vi "Pipe Var Intf - Read Variable - Complex Double.vi"(8 "error in (no error)":errorcluster, 9 "max dims (0: scalar)":i32, 10 "variable name":string, 11 "GOLPI ref. in":T1={"pipe handle"={"lv_proc.dll file path"=path "", "process instance handle"=[], "debug mode"=FALSE, "debug data"=[]}, "fast read timeout [ms]"=500, "fast read settle time [ms]"=10, "fast read to multiple [ms]"=1, "max elements per input line"=100, "slow read timeout [ms]"=5000, "stdin double format specifier"="%_16e", "max elements per stdout output column"=100, "console mode bitstream"=FALSE, "bitstream first read timeout [ms]"=1000, "bitstream read timeout [ms]"=50, "struct transfer possible"=FALSE, "matlab mode"=FALSE, "var pipe write timeout [ms]"=5000, "variable pipe mode"=FALSE, "variable pipe buffer size [Bytes]"=10000000, "variable pipe block size [Bytes]"=1000000} {"variable pipe block size [Bytes]" format="%.0p"; "variable pipe buffer size [Bytes]" format="%.0p"}) -> (0 "error out":errorcluster, 2 "data out":cdb[][](array[numeric]), 3 "GOLPI ref. out":T1={"pipe handle"={"lv_proc.dll file path"=path "", "process instance handle"=[], "debug mode"=FALSE, "debug data"=[]}, "fast read timeout [ms]"=500, "fast read settle time [ms]"=10, "fast read to multiple [ms]"=1, "max elements per input line"=100, "slow read timeout [ms]"=5000, "stdin double format specifier"="", "max elements per stdout output column"=100, "console mode bitstream"=FALSE, "bitstream first read timeout [ms]"=1000, "bitstream read timeout [ms]"=50, "struct transfer possible"=FALSE, "matlab mode"=FALSE, "var pipe write timeout [ms]"=5000, "variable pipe mode"=FALSE, "variable pipe buffer size [Bytes]"=10000000, "variable pipe block size [Bytes]"=1000000} {"variable pipe block size [Bytes]" format="%.0p"; "variable pipe buffer size [Bytes]" format="%.0p"})   [LabVIEW 2020, in "GOLPI library.lvlib"]
doc: "Read matrix from Octave using pipe variable interface. In case of compatible non-doubles, casts to double. max dims defines maximum expected dimensions count."
uses:
  GOLPI library.lvlib
  Public/GOLPI reference Type Def.ctl
  LV Process source distribution/Pipe Handle.ctl
  <vilib>/Utility/error.llb/Error Cluster From Error Code.vi
  <vilib>/ErrorRing/Error Ring.xnode
  LV Process source distribution/LV Process library.lvlib
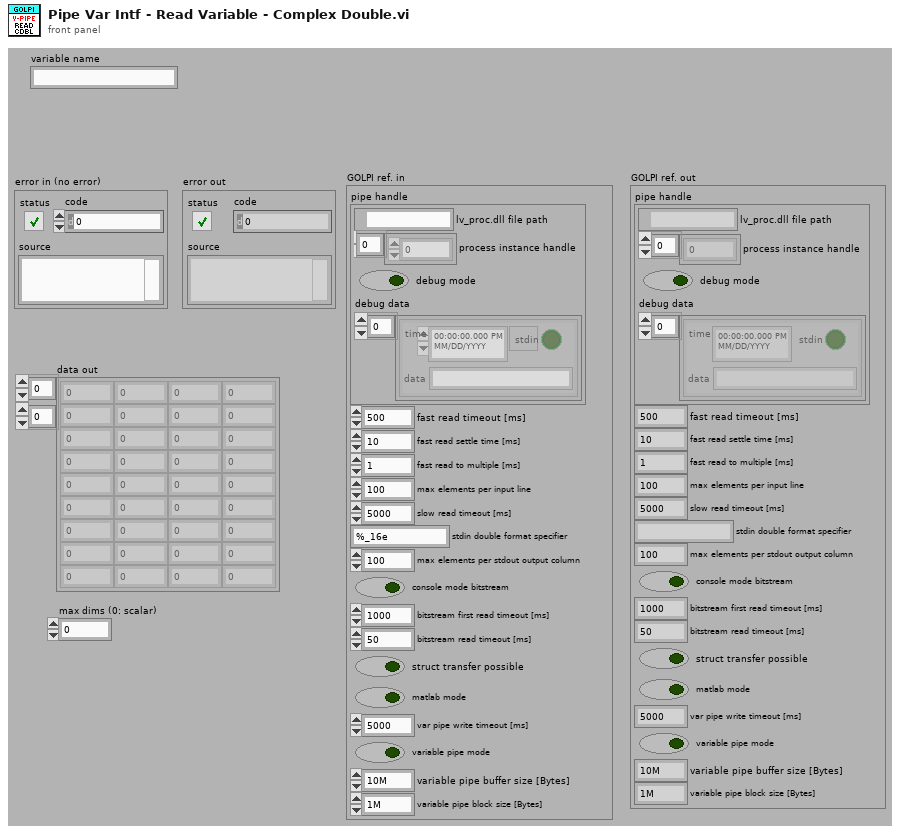
[diagram p1: front panel]
types:
  T1 = typedef "GOLPI library.lvlib/GOLPI reference Type Def.ctl" = cluster{"pipe handle":T2, "fast read timeout [ms]":u32, "fast read settle time [ms]":u32, "fast read to multiple [ms]":u32, "max elements per input line":u32, "slow read timeout [ms]":u32, "stdin double format specifier":string, "max elements per stdout output column":u32, "console mode bitstream":bool, "bitstream first read timeout [ms]":u32, "bitstream read timeout [ms]":u32, "struct transfer possible":bool, "matlab mode":bool, "var pipe write timeout [ms]":u32, "variable pipe mode":bool, "variable pipe buffer size [Bytes]":u32, "variable pipe block size [Bytes]":u32}
  T2 = typedef "LV Process library.lvlib/Pipe Handle.ctl" = cluster{"lv_proc.dll file path":path, "process instance handle":u32[], "debug mode":bool, "debug data":cluster{"time":timestamp, "stdin":bool, "data":string}[]}
  T3 = typedef "GOLPI library.lvlib/Pipe Var Intf - Data Type.ctl" = enum16{"error", "String", "int32", "uint32", "double", "cplx double", "single", "cplx single"}
  T4 = enum16{"big-endian, network order", "native, host order", "little-endian"}
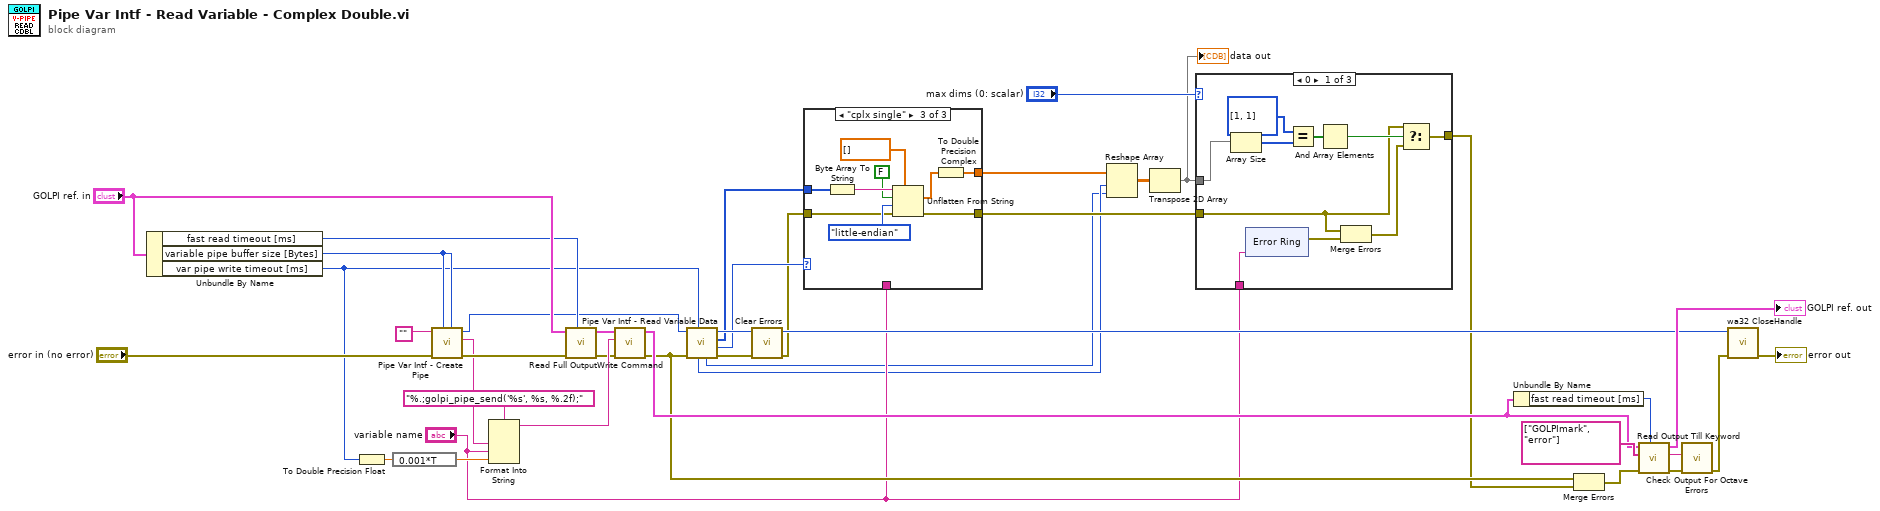
[diagram p0: block diagram]
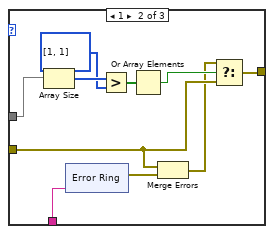
[diagram p2: hidden frame]
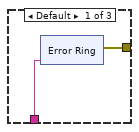
[diagram p4: hidden frame]
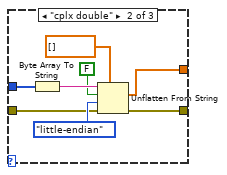
[diagram p5: hidden frame]
diagram:
  n1 = Unbundle By Name("GOLPI ref. in") -> ("fast read timeout [ms]"=w21:u32, "variable pipe buffer size [Bytes]"=w36:u32, "var pipe write timeout [ms]"=w16:u32)
  n2 = To Double Precision Float(number=w16) -> (double precision float=w34:dbl)
  n3 = expression code="0.001*T"(w34) -> (w35:dbl)
  n4 = call "Pipe Var Intf - Create Pipe.vi"("outBufferSize (256k)"=w36, "inBufferSize (256k)"=w36, "error in (no error)"="error in (no error)", "pipe name in (leave empty to generate random name)"="") -> ("error out"=w24:errorcluster, "pipe name out"=w18:string, "pipe handle out"=w17:i32)  [unwired: 5 in]
  n5 = Format Into String(format string="%.;golpi_pipe_send('%s', %s, %.2f);", w18, "variable name", w35) -> (resulting string=w38:string)  [unwired: 2 in, 1 out]
  n6 = call "Read Full Output.vi"("timeout [ms]"=w21, "error in"=w24, "GOLPI ref. in"="GOLPI ref. in") -> ("error out"=w25:errorcluster, "GOLPI ref. out"=w22:T1)  [unwired: 5 in, 2 out]
  n7 = call "Write Command.vi"("error in"=w25, "command"=w38, "GOLPI ref. in"=w22) -> ("error out"=w13:errorcluster, "GOLPI ref. out"=w26:T1)  [unwired: 7 in]
  n8 = call "Pipe Var Intf - Read Variable Data.vi"("timeout [ms]"=w16, "error in (no error)"=w13, "pipe handle"=w17) -> ("error out"=w15:errorcluster, "data type"=w12:T3, "data out"=w11:u8[], "pipe handle out"=w14:i32, "rows"=w2:i32, "columns"=w3:i32)  [unwired: 3 in]
  n9 = call <vilib>:"Clear Errors.vi"("error in (no error)"=w15) -> ("error out"=w10:errorcluster)  [unwired: 5 in, 1 out]
  n10 = case shown="\"cplx single\"" w12 {
    tunnel: w11 -> [_ w52 w61]
    tunnel: w10 -> [_ w51 w60]
    tunnel: [w41 w49 w58] -> w8
    tunnel: "variable name" -> [w40 _ _]
    tunnel: [_ w50 w57] -> w4
    frame Default {
      n11 = xnode "Error Ring"("parameter 0"=w40) -> ("error out"=w41:errorcluster)
    }
    frame "cplx double" {
      n12 = Byte Array To String(unsigned byte array=w52) -> (string=w56:string)
      n13 = Unflatten From String(type=cdb[] [], binary string=w56, data includes array or string size? (T)=FALSE, byte order (0:big-endian, network order)=T4."little-endian", error in (no error)=w51) -> (value=w50:cdb[], error out=w49:errorcluster)  [unwired: 1 out]
    }
    frame "cplx single" {
      n14 = Byte Array To String(unsigned byte array=w61) -> (string=w65:string)
      n15 = Unflatten From String(type=csg[] [], binary string=w65, data includes array or string size? (T)=FALSE, byte order (0:big-endian, network order)=T4."little-endian", error in (no error)=w60) -> (value=w59:csg[], error out=w58:errorcluster)  [unwired: 1 out]
      n16 = To Double Precision Complex(1:w59) -> (0:w57:cdb[])
    }
  }
  n17 = Reshape Array(w4, w3, w2) -> (w5:cdb[][])
  n18 = Transpose 2D Array(2D array=w5) -> (transposed array=w1:cdb[][])
  "data out" <- w1
  n19 = case shown="0" "max dims (0: scalar)" {
    tunnel: w1 -> [w75 w92 _]
    tunnel: w8 -> [w67 w84 w100]
    tunnel: [w70 w91 w100] -> w7
    tunnel: "variable name" -> [w69 w90 _]
    frame 0 {
      n20 = Array Size(array=w75) -> (size(s)=w74:i32[])
      n21 = xnode "Error Ring"("parameter 0"=w69) -> ("error out"=w68:errorcluster)
      n22 = Equal?(x=i32[] [1, 1], y=w74) -> (x = y?=w72:bool[])
      n23 = And Array Elements(Boolean array=w72) -> (logical AND=w71:bool)
      n24 = Merge Errors(w67, w68) -> (w66:errorcluster)
      n25 = Select(t=w67, s=w71, f=w66) -> (s? t:f=w70:errorcluster)
    }
    frame 1 {
      n26 = Array Size(array=w92) -> (size(s)=w88:i32[])
      n27 = xnode "Error Ring"("parameter 0"=w90) -> ("error out"=w89:errorcluster)
      n28 = Greater?(x=w88, y=i32[] [1, 1] ("x")) -> (0:w86:bool[])
      n29 = Or Array Elements(Boolean array=w86) -> (logical OR=w85:bool)
      n30 = Merge Errors(w84, w89) -> (w83:errorcluster)
      n31 = Select(t=w83, s=w85, f=w84) -> (s? t:f=w91:errorcluster)
    }
    frame Default {
    }
  }
  n32 = Unbundle By Name(w26) -> ("fast read timeout [ms]"=w32:u32)
  n33 = Merge Errors(w13, w7) -> (w20:errorcluster)
  n34 = call "Read Output Till Keyword.vi"("timeout [ms]"=w32, "error in"=w20, "keywords"=string[] ["GOLPImark", "error"], "GOLPI ref. in"=w26) -> ("error out"=w31:errorcluster, "read buffer"=w30:string, "GOLPI ref. out"=→"GOLPI ref. out":T1)  [unwired: 4 in, 1 out]
  n35 = call "Check Output For Octave Errors.vi"("error in"=w31, "read buffer"=w30) -> ("error out"=w27:errorcluster)  [unwired: 9 in]
  n36 = call "wa32 CloseHandle.vi"("error in"=w27, "handle"=w14) -> ("error out"=→"error out":errorcluster)  [unwired: 9 in]
